vi "Assert 1D to Data Type.vi"(8 "error in (no error)":errorcluster, 11 "Assert 1D":refnum<class "Assert.lvclass">[](array[class])) -> (0 "error out":errorcluster, 3 "Boolean out":refnum<class "Assertion 1D.lvclass">)   [LabVIEW 2020, in "Assertion 1D.lvclass"]
uses:
  <vilib>/gpm_packages/@cs/data-type-serializer/source/Assertion 1D/Assertion 1D.lvclass
  <vilib>/gpm_packages/@cs/run-time-assertions/Source/Assert/Assert.lvclass
  <vilib>/gpm_packages/@cs/data-type-serializer/source/Assertion 1D/Assertion 1D.lvclass/Assertion 1D.ctl
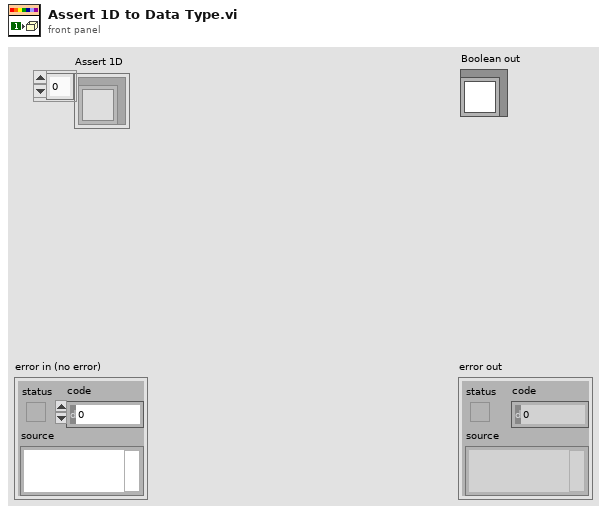
[diagram p1: front panel]
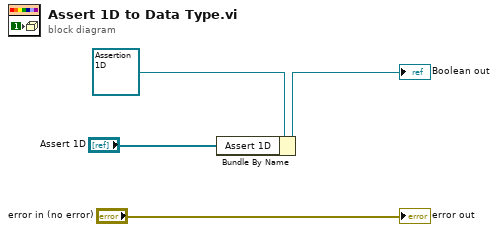
[diagram p0: block diagram]
diagram:
  n1 = Bundle By Name(cluster=refnum<class "Assertion 1D.lvclass"> refnum ("Boolean in"), "Assert 1D"="Assert 1D") -> (→"Boolean out":refnum<class "Assertion 1D.lvclass">)
  "error out" <- "error in (no error)"
